vi "Write id.vi"(8 "error in (no error)":errorcluster, 10 "id":string, 11 "SVG Object in":refnum<class "SVG Object.lvclass">) -> (0 "error out":errorcluster, 3 "SVG Object out":refnum<class "SVG Object.lvclass">)   [LabVIEW 2019, in "SVG Object.lvclass"]
uses:
  SVG Object.lvclass
  SVG Object.lvclass/SVG Object.ctl
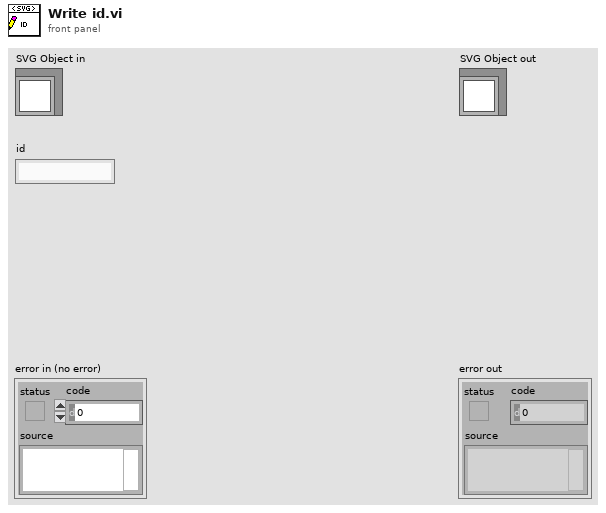
[diagram p1: front panel]
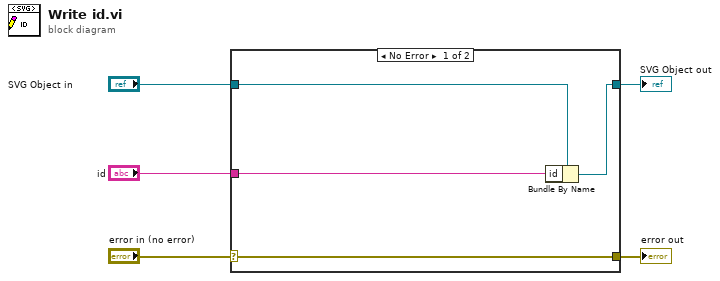
[diagram p0: block diagram]
diagram:
  n1 = case shown="No Error" "error in (no error)" {
    selector: "error in (no error)" -> [w9 w10]
    tunnel: [w9 w10] -> w4
    tunnel: [w7 w11] -> w2
    tunnel: "SVG Object in" -> [w8 w11]
    tunnel: "id" -> [w6 _]
    frame No Error {
      n2 = Bundle By Name(cluster=w8, "id"=w6) -> (w7:refnum<class "SVG Object.lvclass">)
    }
    frame Error {
    }
  }
  "error out" <- w4
  "SVG Object out" <- w2
